vi "Log Data.vi"(8 "error in":errorcluster, 10 "Data":dbl[](array[numeric]), 11 "CSV in":refnum<class "CSV.lvclass">) -> (0 "error out":errorcluster, 3 "CSV out":refnum<class "CSV.lvclass">)   [LabVIEW 2020, in "Manejador archivo.lvlib" / "CSV.lvclass"]
uses:
  CSV.lvclass
  C:/GitClones/DQMH-LabVIEW-GYM/10 Mayo/04 DQMH USER/Libraries/Manejador archivo/Class Definitions/File/File.lvclass
  File/File.lvclass/File.ctl
  CSV.lvclass/CSV.ctl
  File/Read Delimiter.vi
  Read file Ref.vi
  File/Read Save Timestamp.vi
  Write file Ref.vi
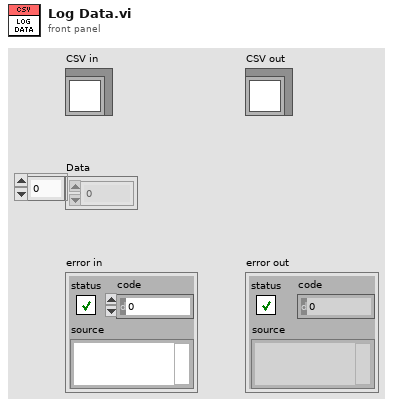
[diagram p1: front panel]
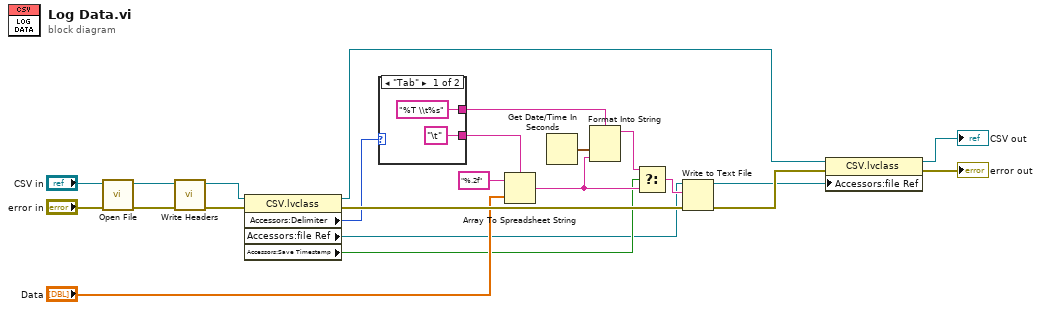
[diagram p0: block diagram]
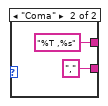
[diagram p2: hidden frame]
diagram:
  n1 = call-dynamic "Open File.vi"("error in"="error in", "CSV in"="CSV in") -> ("error out"=w19:errorcluster, "CSV out"=w6:refnum<class "CSV.lvclass">)  [unwired: 8 in]
  n2 = call "Write Headers.vi"("error in"=w19, "CSV in"=w6) -> ("error out"=w20:errorcluster, "CSV out"=w10:refnum<class "CSV.lvclass">)  [unwired: 8 in]
  n3 = property class="CSV.lvclass"(reference=w10, error in=w20) -> (reference out=w3:refnum<class "CSV.lvclass">, error out=w22:errorcluster, "Accessors:Delimiter"=w7:enum16{"Tab", "Coma"}, "Accessors:file Ref"=w8:refnum<file>, "Accessors:Save Timestamp"=w12:bool)
  n4 = case shown="\"Tab\"" w7 {
    tunnel: ["%T \\t%s" ("format string") "%T ,%s" ("format string")] -> w14
    tunnel: ["\t" ","] -> w9
    frame "Tab" {
    }
    frame "Coma" {
    }
  }
  n5 = Array To Spreadsheet String(delimiter (Tab)=w9, array="Data", 3:"%.2f" ("format string")) -> (spreadsheet string=w16:string)
  n6 = Get Date/Time In Seconds() -> (seconds since 1Jan1904=w18:timestamp)
  n7 = Format Into String(format string=w14, w18, w16) -> (resulting string=w17:string)  [unwired: 2 in, 1 out]
  n8 = Select(t=w17, s=w12, f=w16) -> (s? t:f=w11:string)
  n9 = Write to Text File(file (use dialog)=w8, text=w11, error in=w22) -> (refnum out=w1:refnum<file>, error out=w21:errorcluster)  [unwired: 1 in, 1 out]
  n10 = property class="CSV.lvclass"(reference=w3, error in=w21, "Accessors:file Ref"=w1) -> (reference out=→"CSV out":refnum<class "CSV.lvclass">, error out=→"error out":errorcluster)
